vi "Actor Core.vi"(8 "error in":errorcluster, 11 "RootModelPublishesDoubleFloatX in":refnum<class "ModelSubscribesToDoubleFloatX.lvclass">) -> (0 "error out":errorcluster, 3 "Actor out":refnum<class "Actor.lvclass">)   [LabVIEW 2020, in "ModelSubscribesToDoubleFloatX.lvclass"]
doc: "(<B>Filename</B>: Actor Framework.lvlib:Actor.lvclass:Actor Core.vi)\n\nReceives messages to the actor, reacts to them, and initiates any error handling that may shut the actor down.\n\nDescendant classes may override this VI to append parallel tasks for the actor to complete while it handles messages. Overrides use the Call Parent Method node."
uses:
  ModelSubscribesToDoubleFloatX.lvclass
  ModelSubscribesToDoubleFloatX.lvclass/ModelSubscribesToDoubleFloatX.ctl
  Source/IObserver/IObserver/IObserver.lvclass
  Source/IModel/IModel/IModel.lvclass
  C:/Git/mva-core/Source/IModel/IModel/IModel.lvclass
  C:/Git/mva-core/Source/IObserver/IObserver/IObserver.lvclass
  C:/Program Files (x86)/National Instruments/LabVIEW 2020/vi.lib/ActorFramework/Actor/Actor.lvclass
  C:/Git/mva-core/Test/Doubles/ModelSubscribesToDoubleFloatX/ModelSubscribesToDoubleFloatX.lvclass
  <vilib>/ActorFramework/Actor/Actor.lvclass
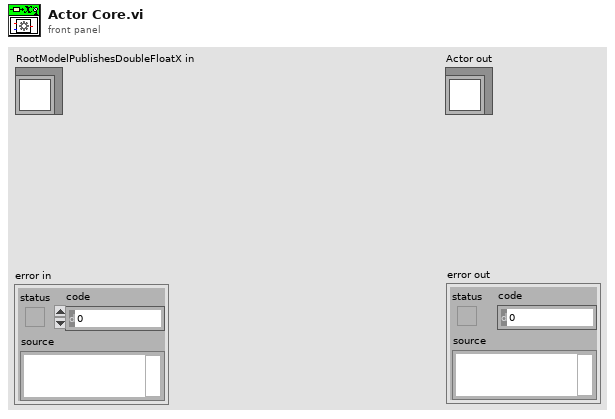
[diagram p1: front panel]
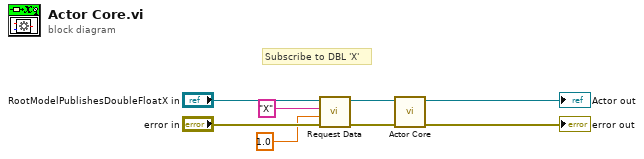
[diagram p0: block diagram]
diagram:
  # "Subscribe to DBL 'X'"
  n1 = call "Request Data.vi"("error in (no error)"="error in", "Data Type"=1.0, "Datum Name"="X", "IObserver in"="RootModelPublishesDoubleFloatX in") -> ("error out"=w5:errorcluster, "IObserver out"=w3:refnum<class "ModelSubscribesToDoubleFloatX.lvclass">)  [unwired: 5 in, 1 out]
  n2 = call-parent "Actor Core.vi"("error in"=w5, "Actor in"=w3) -> ("error out"=→"error out":errorcluster, "Actor out"=→"Actor out":refnum<class "Actor.lvclass">)  [unwired: 8 in]
